vi "SendConnectionModeMessage.vi"() -> ()   [LabVIEW 2011]
uses:
  Shared/J1939 Multi Packet Frame/_SubVIs/CAN Outgoing Message Cluster.ctl
  Shared/J1939 Multi Packet Frame/J1939 Utilities/_SubVIs/Convert CAN Arb ID to J1939 ID.vi
  Shared/J1939 Multi Packet Frame/J1939 Utilities/_SubVIs/J1939 Message TP.CM EndofMsgACK.vi
  Shared/J1939 Multi Packet Frame/J1939 Utilities/_SubVIs/J1939 Message TP.CM RTS.vi
  Shared/J1939 Multi Packet Frame/J1939 Utilities/_SubVIs/J1939 Message TP.DT.vi
  Shared/J1939 Multi Packet Frame/J1939 Utilities/_SubVIs/J1939 Message TP.CM CTS.vi
  Shared/J1939 Multi Packet Frame/J1939 Utilities/_SubVIs/Convert J1939 ID to CAN Arb ID.vi
  <vilib>/NI Veristand/Execution/Workspace/NI VeriStand - Set Single Channel Value.vi
  J1939 Custom Device.lvlib
  Built/Host Automation API/J1939 Host Automation API.lvlibp
  <vilib>/NI Veristand/Execution/Workspace/NI_VS Workspace ExecutionAPI.lvlib
panel:
  out "Expected Value":dbl=84.75123369479934
  out "error out":errorcluster
  in  "Allow Any SA":bool=TRUE
  in  "Data to Send":T1={"Identifier"=469958142, "Data"=[1, 2, 3, 4, 7, 0, 0, 0, 9, 10, 11, 12, 13, 14, 15, 16]} {"Identifier" format="%08x"}
  in  "Source Address":u8
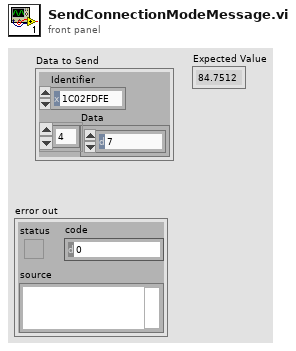
[diagram p1: front panel]
types:
  T1 = typedef "J1939 Custom Device.lvlib/CAN Outgoing Message Cluster.ctl" = cluster{"Identifier":u32, "Data":u8[]}
  T2 = typedef "J1939 Custom Device.lvlib/J1939 PGN Fields Cluster.ctl" = cluster{"Reserved Bit":u8, "Data page":u8, "PDU Format":u8, "PDU Specific":u8}
  T3 = typedef "NI_VS Workspace ExecutionAPI.lvlib/WorkspaceAPI.ctl" = refnum<k24>
  T4 = typedef "J1939 Host Automation API.lvlibp/J1939 Custom Device.lvlib/J1939_stm_TCP Connection Info.ctl" = cluster{"connection ID":refnum<k5>, "Meta data":T5[]}
  T5 = typedef "J1939 Host Automation API.lvlibp/J1939 Custom Device.lvlib/J1939_stm_MetaDataElement.ctl" = string
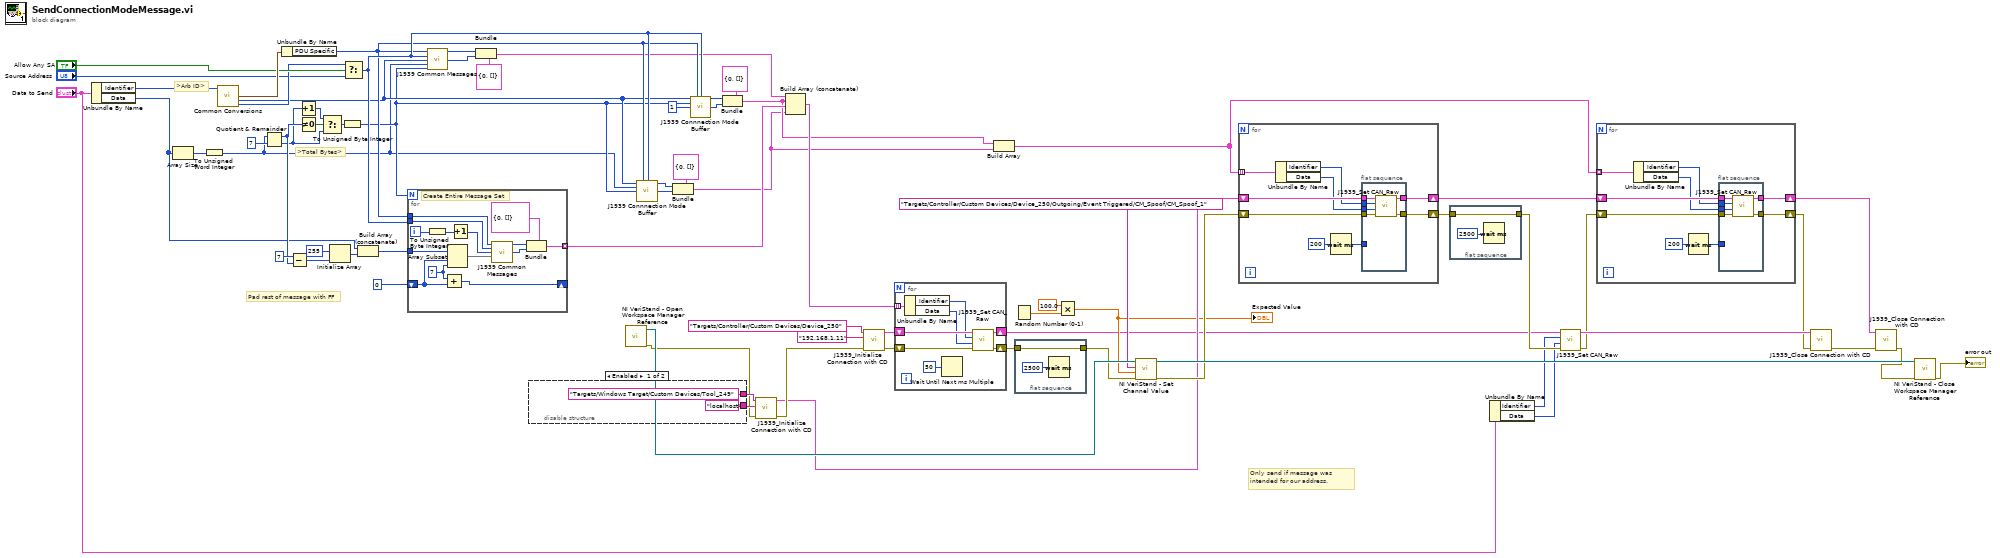
[diagram p0: block diagram]
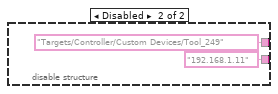
[diagram p2: hidden frame]
diagram:
  # "Only send if message was intended for our address."
  # "Pad rest of message with FF"
  # ">Arb ID>"
  # ">Total Bytes>"
  n1 = Unbundle By Name("Data to Send") -> ("Identifier"=w52:u32, "Data"=w50:u8[])
  n2 = Array Size(array=w50) -> (size(s)=w55:i32)
  n3 = To Unsigned Word Integer(number=w55) -> (unsigned 16bit integer=w37:u16)
  n4 = call-poly "Common Conversions.vi"("Arb ID"=w52) -> ("PGN Fields"=w68:T2, "PGN"=w41:u32, "Source Address"=w48:u8)  [unwired: 12 out]
  n5 = Quotient & Remainder(x=w37, y=u16 7) -> (x-y*floor(x/y)=w63:u16, floor(x/y)=w59:u16)
  n6 = Unbundle By Name(w68) -> ("PDU Specific"=w42:u8)
  n7 = Subtract(x=u8 7, y=w63) -> (x-y=w65:u16)
  n8 = Increment(x=w59) -> (x+1=w58:u16)
  n9 = Not Equal To 0?(x=w63) -> (x != 0?=w57:bool)
  n10 = Select(t=w58, s=w57, f=w59) -> (s? t:f=w60:u16)
  n11 = Initialize Array(u8 255, w65) -> (w66:u8[])
  n12 = To Unsigned Byte Integer(number=w60) -> (unsigned 8bit integer=w40:u8)
  n13 = Select(t=w48, s="Allow Any SA", f="Source Address") -> (s? t:f=w43:u8)
  n14 = Build Array (concatenate)(w50, w66) -> (w67:u8[])
  n15 = for {
    N: w40 -> [_]
    tunnel: w67 -> [w86]
    shift-right: [w83] -> _
    shift-left: 0 ("index") -> [w84]
    tunnel: [w74] -> w38 mode=indexing
    tunnel: w43 -> [w79]
    tunnel: w42 -> [w80]
    i -> [w82]
    w85 = 7 ("length")
    # "Create Entire Message Set"
    n16 = To Unsigned Byte Integer(number=w82) -> (unsigned 8bit integer=w81:u8)
    n17 = Add(x=w85, y=w84) -> (x+y=w83:i32)
    n18 = Array Subset(array=w86, index=w84, length=w85) -> (w77:u8[])
    n19 = Increment(x=w81) -> (x+1=w78:u8)
    n20 = call-poly "J1939 Common Messages.vi"("Destination Address"=w80, "Source Address"=w79, "Sequence Number"=w78, "Data"=w77) -> ("Arb ID"=w76:u32, "Data"=w75:u8[])  [unwired: 10 out]
    n21 = Bundle(cluster=T1 {"Identifier"=0, "Data"=[]}, "Identifier"=w76, "Data"=w75) -> (w74:T1)
  }
  n22 = call-poly "J1939 Common Messages.vi"("Destination Address"=w42, "Source Address"=w43, "PGN"=w41, "Total Message Size(bytes)"=w37, "Total Number of Packets"=w40) -> ("Arb ID"=w54:u32, "Data"=w53:u8[])  [unwired: 9 out]
  n23 = Bundle(cluster=T1 {"Identifier"=0, "Data"=[]}, "Identifier"=w54, "Data"=w53) -> (w39:T1)
  n24 = disable-structure shown="Enabled" {
    disable-tunnel: ["Targets/Windows Target/Custom Devices/Tool_249" ("Custom Device Path") "Targets/Controller/Custom Devices/Tool_249" ("Custom Device Path")] -> w22
    disable-tunnel: ["localhost" ("Unit Computer Address") "192.168.1.11" ("Unit Computer Address")] -> w21
    frame Enabled {
    }
    frame Disabled {
    }
  }
  n25 = call <vilib>:"NI VeriStand - Open Workspace Manager Reference.vi"() -> ("error out"=w20:errorcluster, "WorkspaceManager"=w31:T3)  [unwired: 10 in]
  n26 = call-poly "J1939 Connnection Mode Buffer.vi"("PGN"=w41, "Source Address"=w42, "Destination Address"=w43, "Total Message Size(bytes)"=w37, "Total Number of Packets"=w40) -> ("Arb ID"=w46:u32, "Data"=w45:u8[])  [unwired: 1 in, 8 out]
  n27 = Bundle(cluster=T1 {"Identifier"=0, "Data"=[]} ("Data to Send"), "Identifier"=w46, "Data"=w45) -> (w24:T1)
  n28 = call-poly "J1939 Connnection Mode Buffer.vi"("PGN"=w41, "Source Address"=w42, "Destination Address"=w43, "Number of Packets to Send"=w40, "Next Packet to Send"=u8 1) -> ("Arb ID"=w71:u32, "Data"=w70:u8[])  [unwired: 2 in, 7 out]
  n29 = Bundle(cluster=T1 {"Identifier"=0, "Data"=[]} ("Data to Send"), "Identifier"=w71, "Data"=w70) -> (w25:T1)
  n30 = call "J1939_Initialize Connection with CD.vi"("error in (no error)"=w20, "Unit Computer Address"=w21, "Custom Device Path"=w22) -> ("error out"=w19:errorcluster, "Connection Info"=w18:T4)  [unwired: 6 in, 1 out]
  n31 = Build Array (concatenate)(w39, w25, w38, w24) -> (w34:T1[])
  n32 = call "J1939_Initialize Connection with CD.vi"("error in (no error)"=w19, "Unit Computer Address"="192.168.1.11", "Custom Device Path"="Targets/Controller/Custom Devices/Device_250") -> ("error out"=w35:errorcluster, "Connection Info"=w36:T4)  [unwired: 6 in, 1 out]
  n33 = for {
    shift-right: [w96] -> w30
    shift-left: w35 -> [w95]
    shift-right: [w97] -> w10
    shift-left: w36 -> [w98]
    tunnel: w34 -> [w94] mode=indexing
    n34 = Unbundle By Name(w94) -> ("Identifier"=w92:u32, "Data"=w93:u8[])
    n35 = Wait Until Next ms Multiple(millisecond multiple=u32 50) -> ()  [unwired: 1 out]
    n36 = call "J1939_Set CAN_Raw.vi"("error in (no error)"=w95, "Data"=w93, "Identifier"=w92, "Connection Info"=w98) -> ("error out"=w96:errorcluster, "Connection Info"=w97:T4)  [unwired: 6 in]
  }
  n37 = Build Array(w25, w24) -> (w2:T1[])
  n38 = Random Number (0-1)() -> (number: 0 to 1=w15:dbl)
  n39 = flat-sequence {
    tunnel: [w100] -> w29
    tunnel: w30 -> [w100]
    frame #0 {
      n40 = Wait (ms)(milliseconds to wait=u32 2500) -> ()  [unwired: 1 out]
    }
  }
  n41 = Multiply(x=100.0, y=w15) -> (x*y=w13:dbl)
  "Expected Value" <- w13
  n42 = call-poly <vilib>:"NI VeriStand - Set Channel Value.vi"("error in (no error)"=w29, "Value"=w13, "Channel"="Targets/Controller/Custom Devices/Device_250/Outgoing/Event Triggered/CM_Spoof/CM_Spoof_1" ("Custom Device Path"), "WorkspaceManager in"=w31) -> ("error out"=w23:errorcluster, "WorkspaceManager out"=w27:T3)  [unwired: 6 in]
  n43 = for {
    shift-right: [w107] -> w12
    shift-left: w23 -> [w106]
    shift-right: [w108] -> w5
    shift-left: w18 -> [w109]
    tunnel: w2 -> [w105] mode=indexing
    n44 = Unbundle By Name(w105) -> ("Identifier"=w103:u32, "Data"=w104:u8[])
    n45 = Wait (ms)(milliseconds to wait=u32 200) -> (millisecond timer value=w101:u32)
    n46 = flat-sequence {
      tunnel: w109 -> [w115]
      tunnel: [w114] -> w108
      tunnel: [w113] -> w107
      tunnel: w106 -> [w112]
      tunnel: w104 -> [w111]
      tunnel: w103 -> [w110]
      tunnel: w101 -> [_]
      frame #0 {
        n47 = call "J1939_Set CAN_Raw.vi"("error in (no error)"=w112, "Data"=w111, "Identifier"=w110, "Connection Info"=w115) -> ("error out"=w113:errorcluster, "Connection Info"=w114:T4)  [unwired: 6 in]
      }
    }
  }
  n48 = flat-sequence {
    tunnel: [w117] -> w11
    tunnel: w12 -> [w117]
    frame #0 {
      n49 = Wait (ms)(milliseconds to wait=u32 2500) -> ()  [unwired: 1 out]
    }
  }
  n50 = Unbundle By Name("Data to Send") -> ("Identifier"=w7:u32, "Data"=w6:u8[])
  n51 = call "J1939_Set CAN_Raw.vi"("error in (no error)"=w11, "Data"=w6, "Identifier"=w7, "Connection Info"=w10) -> ("error out"=w3:errorcluster, "Connection Info"=w9:T4)  [unwired: 6 in]
  n52 = for {
    shift-right: [w124] -> w1
    shift-left: w3 -> [w123]
    shift-right: [w125] -> w4
    shift-left: w5 -> [w126]
    tunnel: w2 -> [w122] mode=indexing
    n53 = Unbundle By Name(w122) -> ("Identifier"=w120:u32, "Data"=w121:u8[])
    n54 = Wait (ms)(milliseconds to wait=u32 200) -> (millisecond timer value=w118:u32)
    n55 = flat-sequence {
      tunnel: w126 -> [w132]
      tunnel: [w131] -> w125
      tunnel: [w130] -> w124
      tunnel: w123 -> [w129]
      tunnel: w121 -> [w128]
      tunnel: w120 -> [w127]
      tunnel: w118 -> [_]
      frame #0 {
        n56 = call "J1939_Set CAN_Raw.vi"("error in (no error)"=w129, "Data"=w128, "Identifier"=w127, "Connection Info"=w132) -> ("error out"=w130:errorcluster, "Connection Info"=w131:T4)  [unwired: 6 in]
      }
    }
  }
  n57 = call "J1939_Close Connection with CD.vi"("error in (no error)"=w1, "Connection Info"=w9) -> ("error out"=w17:errorcluster)  [unwired: 9 in]
  n58 = call "J1939_Close Connection with CD.vi"("error in (no error)"=w17, "Connection Info"=w4) -> ("error out"=w16:errorcluster)  [unwired: 9 in]
  n59 = call <vilib>:"NI VeriStand - Close Workspace Manager Reference.vi"("error in (no error)"=w16, "WorkspaceManager"=w27) -> ("error out"=→"error out":errorcluster)  [unwired: 9 in]
